vi "LowSpeedWarningTracepoint.vi"(7 "Qbus in":refnum<class "Qbus.lvclass">, 8 "error in (no error)":errorcluster, 11 "group":T1) -> (0 "error out":errorcluster, 3 "group out":T1)   [LabVIEW 2017]
uses:
  <vilib>/addons/TraceLogger/TraceLogger.lvlib
  <vilib>/addons/Qbus/Qbus.lvclass
  <vilib>/addons/InsightCM/Utilities/Analysis/Shared/controls/AmplitudeScale.ctl
  <vilib>/addons/InsightCM/Utilities/Analysis/Shared/AnalysisHelper.lvlib
  <vilib>/addons/InsightCM/Utilities/Analysis/Shared/controls/Feature.ctl
  <vilib>/addons/InsightCM/Utilities/Analysis/Shared/controls/Channel.ctl
  <vilib>/addons/InsightCM/Devices/Shared/VibrationAnalysis/controls/Group.ctl
  <vilib>/addons/InsightCM/Utilities/Analysis/Shared/controls/SpeedType.ctl
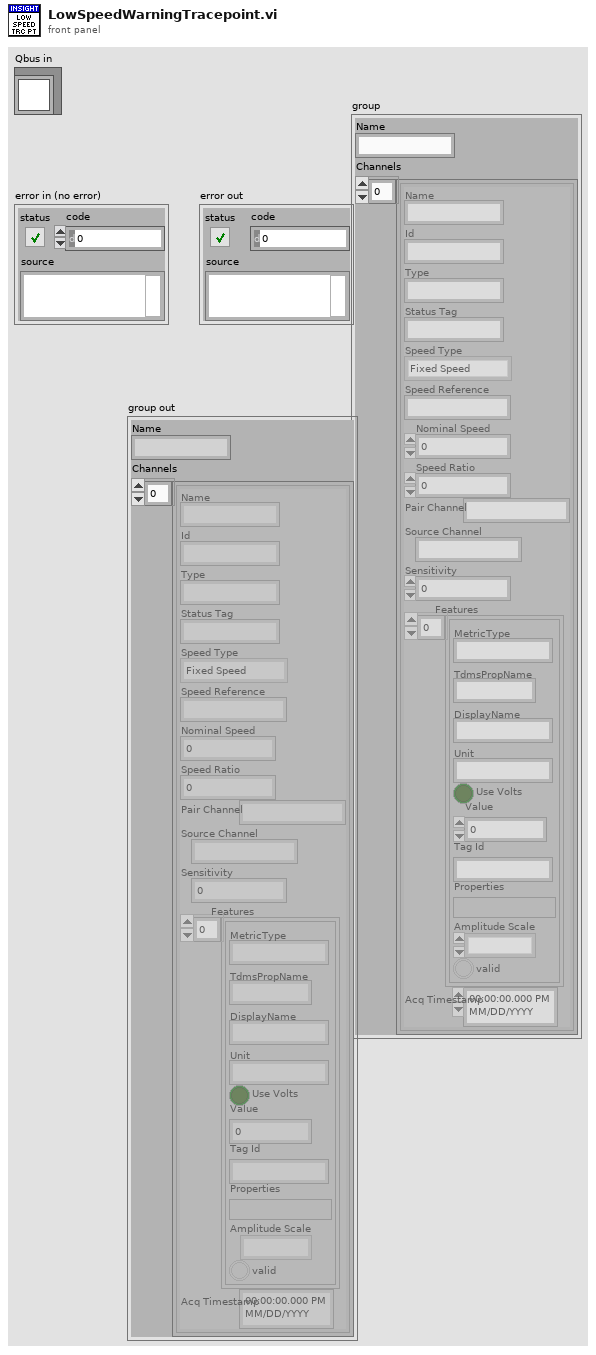
[diagram p1: front panel]
types:
  T1 = typedef "VibrationAnalysis.lvlib/Group.ctl" = cluster{"Name":string, "Channels":T2[]}
  T2 = typedef "AnalysisHelper.lvlib/Channel.ctl" = cluster{"Name":string, "Id":string, "Type":string, "Status Tag":string, "Speed Type":T3, "Speed Reference":string, "Nominal Speed":dbl, "Speed Ratio":dbl, "Pair Channel":string, "Source Channel":string, "Sensitivity":dbl, "Features":T4[], "Acq Timestamp":timestamp}
  T3 = typedef "AnalysisHelper.lvlib/SpeedType.ctl" = enum16{"Fixed Speed", "Tachometer"}
  T4 = typedef "AnalysisHelper.lvlib/Feature.ctl" = cluster{"MetricType":string, "TdmsPropName":string, "DisplayName":string, "Unit":string, "Use Volts":bool, "Value":dbl, "Tag Id":string, "Properties":variant, "Amplitude Scale":T5, "valid":bool}
  T5 = typedef "AnalysisHelper.lvlib/AmplitudeScale.ctl" = enum16{"rms", "peak", "pk-pk"}
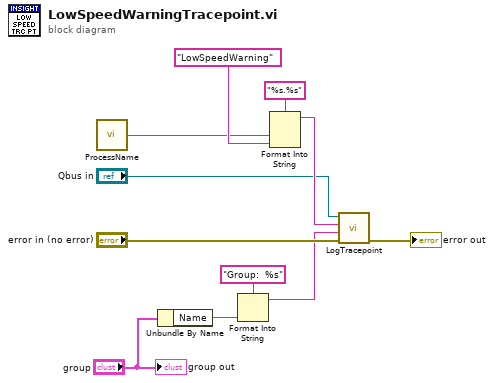
[diagram p0: block diagram]
diagram:
  n1 = call <vilib>:"ProcessName.vi"() -> ("ProcessName"=w3:string)  [unwired: 5 in]
  n2 = Unbundle By Name("group") -> ("Name"=w1:string)
  n3 = Format Into String(format string="Group:  %s", w1) -> (resulting string=w4:string)  [unwired: 2 in, 1 out]
  n4 = Format Into String(format string="%s.%s", w3, "LowSpeedWarning" ("tracepoint")) -> (resulting string=w8:string)  [unwired: 2 in, 1 out]
  n5 = call <vilib>:"LogTracepoint.vi"("error in (no error)"="error in (no error)", "log string"=w4, "tracepoint"=w8, "qbus in"="Qbus in") -> ("error out"=→"error out":errorcluster)  [unwired: 6 in, 1 out]
  "group out" <- "group"
